vi "pwm.vi"() -> ()   [LabVIEW 2016]
panel:
  out "Waveform Graph 2":dynamicdata(graph)
  out "Waveform Graph":dynamicdata(graph)
  in  "Frequency 2":dbl(knob)=10.1 caption="Frequency" scale=0.0..5000.0
  in  "Frequency":dbl(knob)=10.1 scale=0.0..100.0
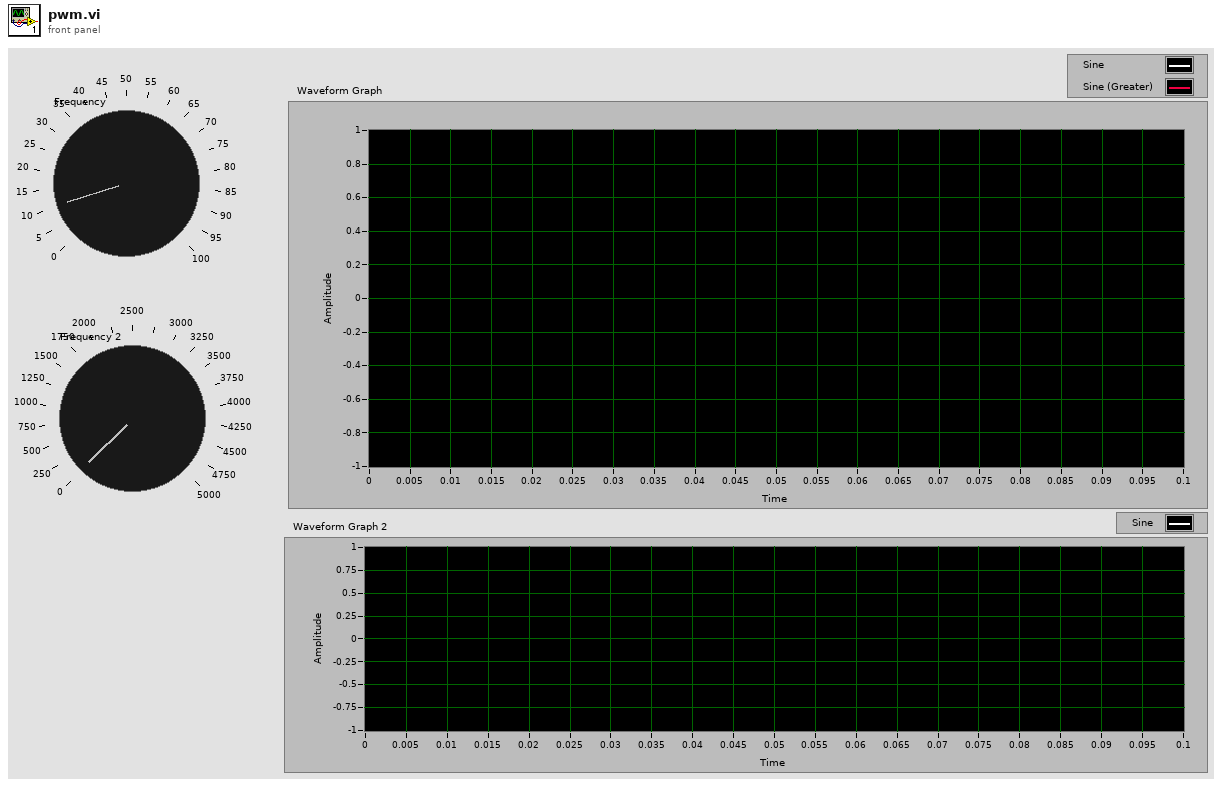
[diagram p1: front panel]
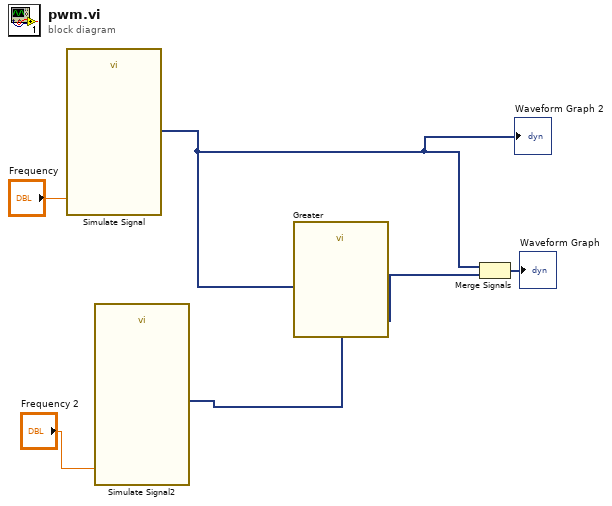
[diagram p0: block diagram]
diagram:
  n1 = call "Simulate Signal"("Frequency"="Frequency") -> ("Sine"=w1:dynamicdata)  [unwired: 13 in, 1 out]
  "Waveform Graph 2" <- w1
  n2 = call "Simulate Signal2"("Frequency"="Frequency 2") -> ("Triangle"=w4:dynamicdata)  [unwired: 13 in, 1 out]
  n3 = call "Greater"("Operand 2"=w4, "Operand 1"=w1) -> ("Result"=w3:dynamicdata)  [unwired: 8 in, 1 out]
  n4 = Merge Signals(w1, w3) -> (→"Waveform Graph":dynamicdata)
